vi "2d angular offset.vi"(8 "Vector 2":dbl[](array[numeric]), 11 "Vector 1":dbl[](array[numeric])) -> (2 "Offset Angle":dbl)   [LabVIEW 2011]
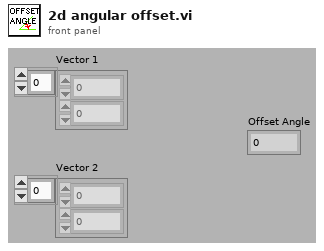
[diagram p1: front panel]
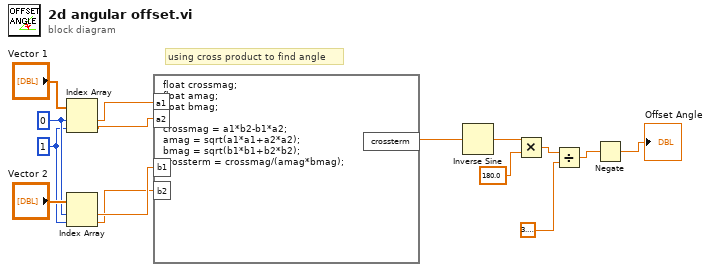
[diagram p0: block diagram]
diagram:
  w12 = 1 ("index")
  w13 = 0 ("index")
  # "using cross product to find angle"
  n1 = Index Array(array="Vector 1", index #1=w13, index #2=w12) -> (element #1=w11:dbl, element #2=w10:dbl)
  n2 = Index Array(array="Vector 2", index #1=w13, index #2=w12) -> (element #1=w9:dbl, element #2=w8:dbl)
  n3 = formula code="float crossmag;\nfloat amag;\nfloat bmag;\n\ncrossmag = a1*b2-b1*a2;\namag = sqrt(a1*a1+a2*a2);\nbmag = sqrt(b1*b1+b2*b2);\ncrossterm = crossmag/(amag*bmag);"("a1"=w11, "a2"=w10, "b1"=w9, "b2"=w8) -> ("crossterm"=w7:dbl)
  n4 = Inverse Sine(1:w7) -> (0:w6:dbl)
  n5 = Multiply(x=w6, y=180.0) -> (x*y=w4:dbl)
  n6 = Divide(x=w4, y=3.141592653589793) -> (x/y=w2:dbl)
  n7 = Negate(x=w2) -> (-x=→"Offset Angle":dbl)
